vi "saveControl.vi"(8 "error in (no error)":errorcluster, 11 "Enumeration in":refnum<class "Enumeration.lvclass">) -> (0 "error out":errorcluster, 3 "Enumeration out":refnum<class "Enumeration.lvclass">)   [LabVIEW 2018, in "Enumeration.lvclass"]
uses:
  Enumeration.lvclass
  Enumeration.lvclass/Enumeration.ctl
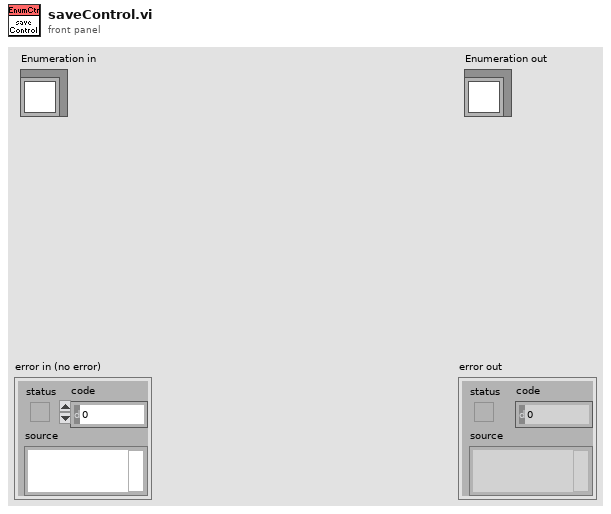
[diagram p1: front panel]
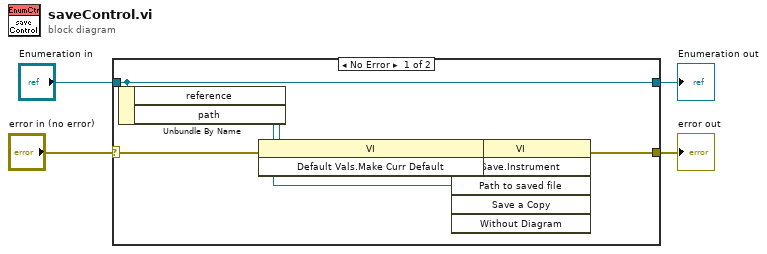
[diagram p0: block diagram]
diagram:
  n1 = case shown="No Error" "error in (no error)" {
    selector: "error in (no error)" -> [w7 w13]
    tunnel: [w5 w13] -> w3
    tunnel: [w6 w12] -> w1
    tunnel: "Enumeration in" -> [w6 w12]
    frame No Error {
      n2 = Unbundle By Name(w6) -> ("reference"=w10:refnum<vi>, "path"=w11:path)
      n3 = invoke class="VI" method="Default Vals.Make Curr Default"(reference=w10, error in=w7) -> (reference out=w8:refnum<vi>, error out=w9:errorcluster)  [unwired: 1 in, 1 out]
      n4 = invoke class="VI" method="Save.Instrument"(reference=w8, error in=w9, "Path to saved file"=w11) -> (error out=w5:errorcluster)  [unwired: 3 in, 5 out]
    }
    frame Error {
    }
  }
  "error out" <- w3
  "Enumeration out" <- w1
